vi "Filter FF_Q.vi"(5 "Reset":bool=TRUE, 8 "input valid":bool=TRUE, 9 "Buffer size":u32, 11 "source adress":u32) -> (0 "output valid":bool)   [LabVIEW 2018]
uses:
  <vilib>/rvi/Memory/Memory_Emulation/nirvimemoryFastEmulation.vi
  <vilib>/rvi/Memory/Memory_Emulation/nirvimemoryEmulation.vi
  <vilib>/rvi/Emulation/niFpgaEmulationIsFPGAContextNoSignature.vi
  <vilib>/rvi/DataTransferAndStorage/Container/Common/niFpgaContainerGetUniqueNameForEmu.vi
  <vilib>/rvi/Emulation/niFpgaProcessEmulError.vi
  <vilib>/rvi/Emulation/niFpgaSctlEmulationGetInTimedLoop.vi
  <vilib>/rvi/errors/nirviReportUnexpectedCaseInternalError (U32).vi
  <vilib>/rvi/DataTransferAndStorage/Container/XNode/niFpgaContainer.xnode
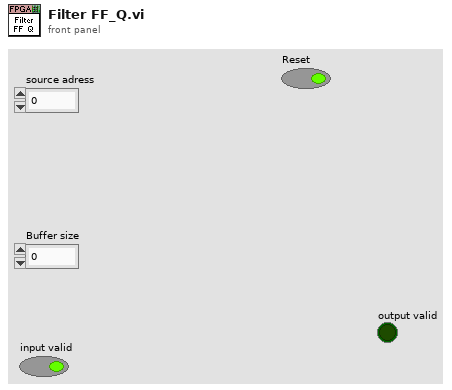
[diagram p1: front panel]
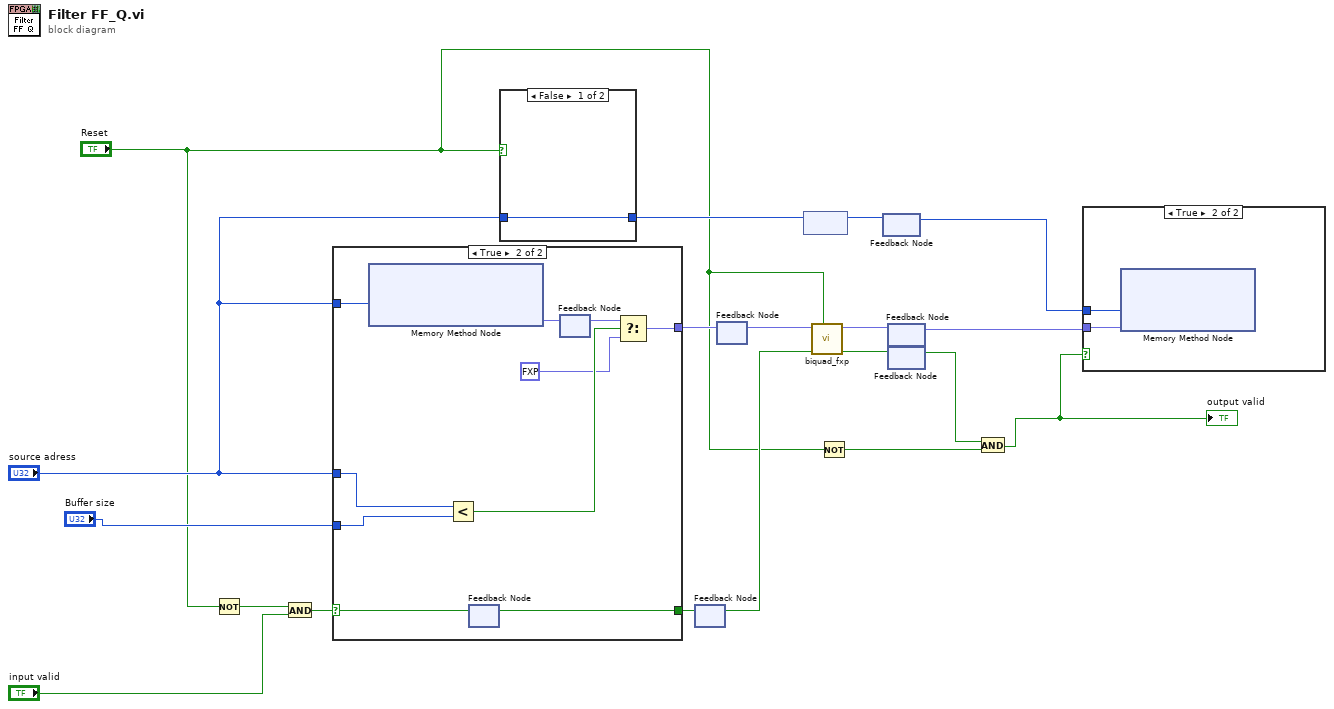
[diagram p0: block diagram]
diagram:
  n1 = Not(x="Reset") -> (.not. x?=w12:bool)
  n2 = And(x=w12, y="input valid") -> (x .and. y?=w13:bool)
  n3 = case shown="True" w13 {
    selector: w13 -> [_ w27]
    tunnel: "source adress" -> [_ w25]
    tunnel: [_ w22] -> w18
    tunnel: "source adress" -> [_ w29]
    tunnel: [_ w26] -> w17
    tunnel: "Buffer size" -> [_ w24]
    frame False {
    }
    frame True {
      n4 = xnode ("Memory Method Node")("Address"=w29) -> ("Data"=w28:fxp<+/-,32,14>)  [unwired: 1 in, 1 out]
      n5 = Less?(x=w25, y=w24) -> (x < y?=w21:bool)
      n6 = feedback #1() -> (w26:bool)  [unwired: 1 in]
      n7 = feedback-in #1(w27) -> ()
      n8 = feedback #2() -> (w23:fxp<+/-,32,14>)  [unwired: 1 in]
      n9 = feedback-in #2(w28) -> ()
      n10 = Select(t=w23, s=w21, f=fxp<+/-,32,14> 0.0) -> (s? t:f=w22:fxp<+/-,32,14>)
    }
  }
  n11 = case shown="False" "Reset" {
    tunnel: "source adress" -> [w30 _]
    tunnel: [w30 _] -> w9
    frame False {
    }
    frame True {
    }
  }
  n12 = feedback #3() -> (w8:bool)  [unwired: 1 in]
  n13 = feedback-in #3(w17) -> ()
  n14 = feedback #4() -> (w11:fxp<+/-,32,14>)  [unwired: 1 in]
  n15 = feedback-in #4(w18) -> ()
  n16 = feedback #5() -> (w6:u32)  [unwired: 1 in]
  n17 = feedback-in #5(w9) -> ()
  n18 = call "biquad_fxp.vi"("reset"="Reset", "input valid"=w8, "x"=w11) -> ("output valid"=w3:bool, "y"=w4:fxp<+/-,32,14>)  [unwired: 7 in]
  n19 = Not(x="Reset") -> (.not. x?=w19:bool)
  n20 = feedback #6() -> (w5:u32)  [unwired: 1 in]
  n21 = feedback-in #6(w6) -> ()
  n22 = feedback #7() -> (w2:fxp<+/-,32,14>)  [unwired: 1 in]
  n23 = feedback-in #7(w4) -> ()
  n24 = feedback #8() -> (w1:bool)  [unwired: 1 in]
  n25 = feedback-in #8(w3) -> ()
  n26 = And(x=w1, y=w19) -> (x .and. y?=w16:bool)
  "output valid" <- w16
  n27 = case shown="True" w16 {
    tunnel: w2 -> [_ w32]
    tunnel: w5 -> [_ w31]
    frame False {
    }
    frame True {
      n28 = xnode ("Memory Method Node")("Address"=w31, "Data"=w32) -> ()  [unwired: 1 in, 1 out]
    }
  }
